vi "NACA_0015_Pressure_with_profile_fixed.vi"(3 "Mode":T5, 5 "Traverse line In":T1 {"Row Duration (mins)" format="%#.1f"; "Row No" min=0; "Trace Gas Concentration (%)" min=0.0 format="%#.2f"; "Emission Rate (l/min)" format="%#.2f"; "Tunnel Speed" format="%#.2f"; "Start X" format="%#.2f"; "Start Y" format="%#.2f"; "Start Z" format="%#.2f"; "End X" format="%#.2f"; "End Y" format="%#.2f"; "End Z" format="%#.2f"; "Averaging time (min)" min=0.0 format="%#.2f"}) -> (0 "Error Message":string, 1 "Status":T4, 2 "Traverse line Out":T1 {"Row Duration (mins)" format="%#.1f"; "Row No" min=0; "Trace Gas Concentration (%)" min=0.0 format="%#.2f"; "Emission Rate (l/min)" format="%#.2f"; "Tunnel Speed" format="%#.2f"; "Start X" format="%#.2f"; "Start Y" format="%#.2f"; "Start Z" format="%#.2f"; "End X" format="%#.2f"; "End Y" format="%#.2f"; "End Z" format="%#.2f"; "Averaging time (min)" min=0.0 format="%#.2f"})   [LabVIEW 2012]
uses:
  Gen Trav/Traverse_cluster.ctl
  Gen Trav/Spacing.ctl
  Controls/Multi_run_mode.ctl
  Controls/User_Specific_mode.ctl
  Gen Trav/Multi_Run_Status.ctl
  Gen Trav/Trav_mode.ctl
  Controls/Setup.ctl
  Controls/Save_Data.ctl
  <vilib>/Analysis/1siggen.llb/Ramp Pattern by Delta.vi
  <vilib>/Analysis/1siggen.llb/Ramp Pattern by Samples.vi
  Globals/Extra_Commands_Global.vi
  Globals/Meas_global.vi
  <vilib>/Analysis/NI_AALBase.lvlib
panel:
  out "Wake Profile":cluster{dbl[], dbl[]}(graph)
  in  "stop":bool
  out "Pressure":cluster{dbl[], dbl[]}(graph)
  out "Measurement No":i32
  # "X           Y            Z"
  # "Start"
  # "End"
  # "X           Y            Z"
  # "Start"
  # "End"
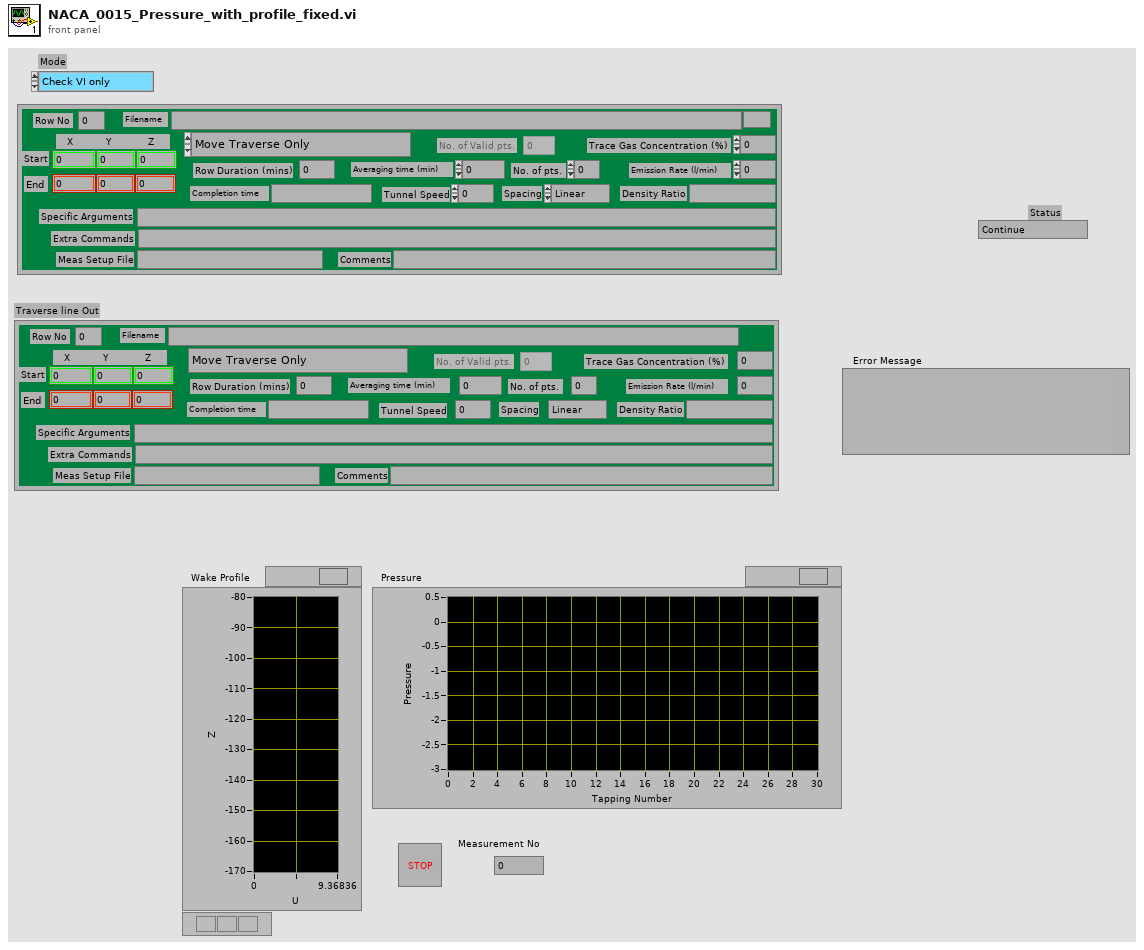
[diagram p1: front panel]
types:
  T1 = typedef "Traverse_cluster.ctl" = cluster{"Start X":dbl, "Start Y":dbl, "Start Z":dbl, "End X":dbl, "End Y":dbl, "End Z":dbl, "No. of pts.":i32, "Spacing":T2, "Filename":path, "Tunnel Speed":dbl, "Averaging time (min)":dbl, "Extra Commands":string, "Specific Arguments":string, "Emission Rate (l/min)":dbl, "Trace Gas Concentration (%)":dbl, "Density Ratio":string, "Comments":string, "Row No":i32, "Row Type Selector":T3, "Completion time":string, "Row Duration (mins)":dbl, "No. of Valid pts.":i32, "Meas Setup File":string}
  T2 = typedef "Spacing.ctl" = enum16{"Linear", "Log", "Gauss", "Specified", "N/A"}
  T3 = typedef "Multi_run_mode.ctl" = enum16{"Move Traverse Only", "Set Tunnel Speed Only", "Set Source Only", "Set Measurement Conditions", "Single Measurement", "Vertical Profile", "Lateral Profile", "Longitudinal Profile", "Explore Volume", "Multi-Axis Profile", "Auto Calibrate", "Meas Fast FID Bkgnd", "Check Beam Power", "Scanning Valve Measurement", "Run VI Named:", "Set ADAM Ch", "Wait (minutes)", "Send Message", "Synchronize With:", "Fall Back to this Row", "Turn Off Row Repeating", "Blank Row", "Traverse 3D Volume"}
  T4 = typedef "Multi_Run_Status.ctl" = enum16{"Continue", "Jump to Next Point", "Jump to Next Row", "Jump To Fall Back", "Terminate Run"}
  T5 = typedef "User_Specific_mode.ctl" = enum16{"Check VI only", "Run VI"}
  T6 = typedef "Trav_mode.ctl" = enum16{"Move traverse", "Read traverse position", "Teach Position"}
  T7 = typedef "Save_Data.ctl" = enum16{"Save No Data", "Save Data"}
  T8 = typedef "Setup.ctl" = enum16{"Run Program", "Show Setup", "Save Current Setup", "Setup Front Panel"}
  T9 = typedef "Status_Cluster.ctl" = cluster{"Status":T4, "Error Type":string, "Error Description":string}
  T10 = typedef "Analysis_info_cluster.ctl" = cluster{"Colour":u32, "Inst type":T11, "Inst name":string, "Symbol":string, "Code name":string, "Extra Info":string, "Inst Array":T12, "Extra Titles":string[], "Extra Values":string[], "U":dbl, "u^2":dbl, "u^3":dbl, "u^4":dbl, "Skew_u":dbl, "Kurt_u":dbl, "Sd Error in Mean":dbl, "% u'/U":dbl, "X":dbl, "Y":dbl, "Z":dbl, "Timescale integral to 25%":dbl, "Sd Error in Variance":dbl, "Calib File":path, "Calib Constants":dbl[], "Output Position":bool, "Full Stats":bool, "Av Sampling Rate":dbl, "Av No of Samples":dbl, "Total Meas Time (s)":dbl, "ADAM Ch Name":string}
  T11 = typedef "Inst_type.ctl" = enum16{"Propeller anemometer", "Raw voltage", "Pressure Transducer", "Pitot-static tube", "Preston tube", "Hot wire", "Cross wire 1", "Cross wire 2", "Generic Linear", "Generic Polynomial", "Generic BackPoly", "Fast FID", "Thermocouple", "Cold wire", "Pulsed Wire", "LDA Vel", "LDA Tran time", "LDA Arr time"}
  T12 = typedef "Instrument_Array.ctl" = enum16{"PWA", "LDA", "Analogue"}
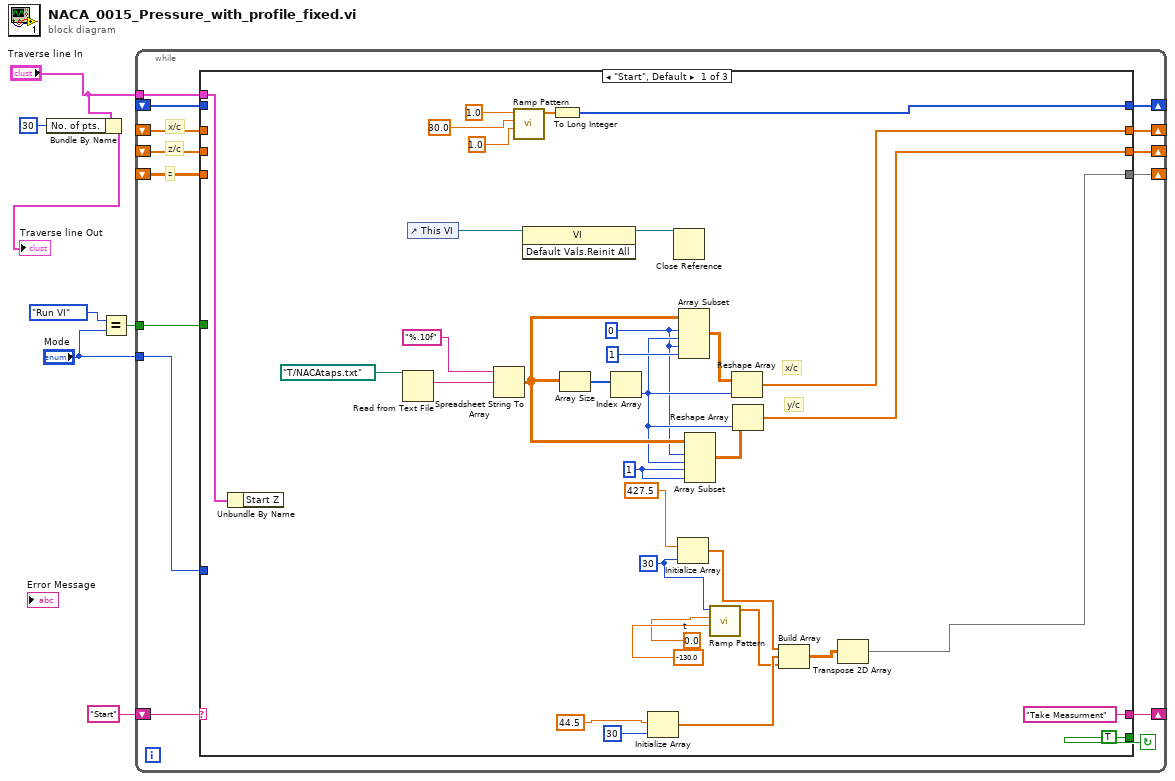
[diagram p0: block diagram]
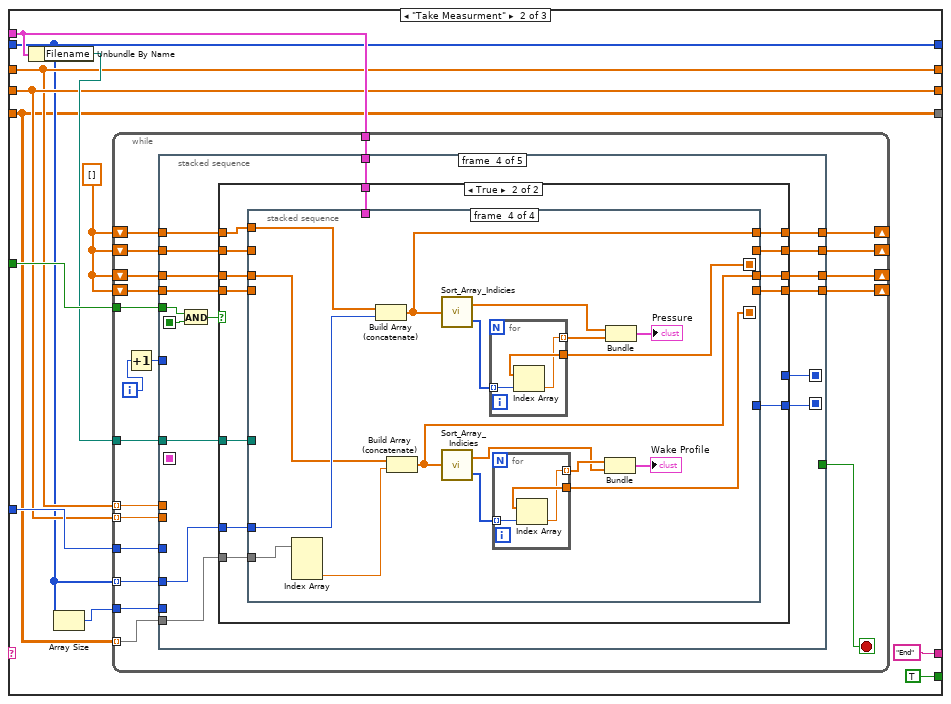
[diagram p2: hidden frame]
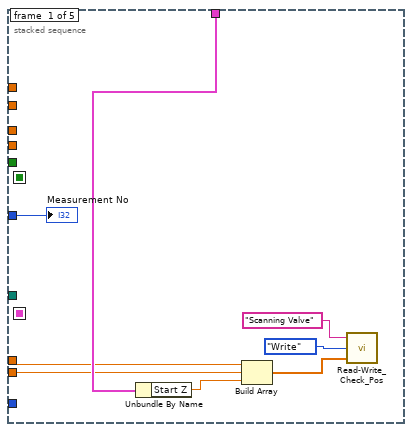
[diagram p3: hidden frame]
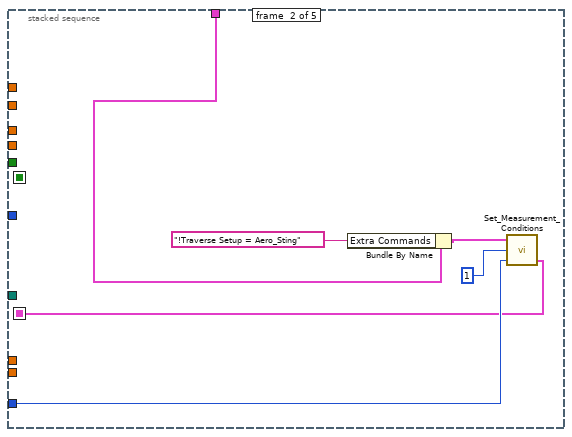
[diagram p4: hidden frame]
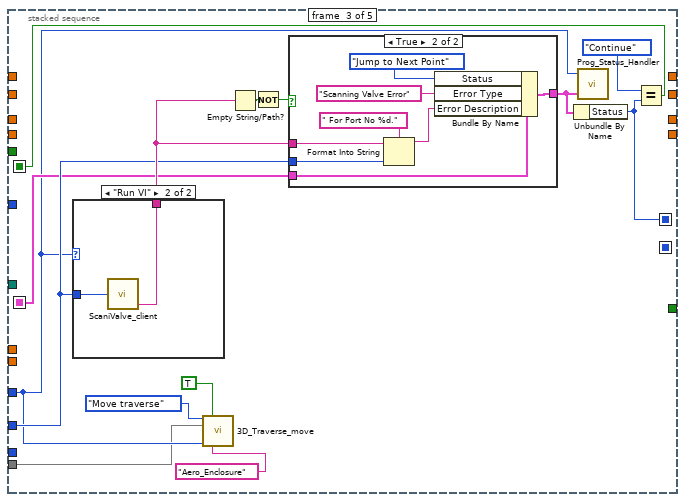
[diagram p5: hidden frame]
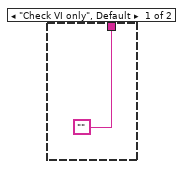
[diagram p6: hidden frame]
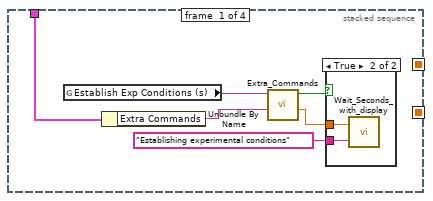
[diagram p9: hidden frame]
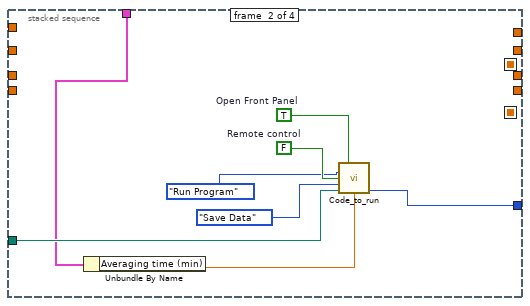
[diagram p11: hidden frame]
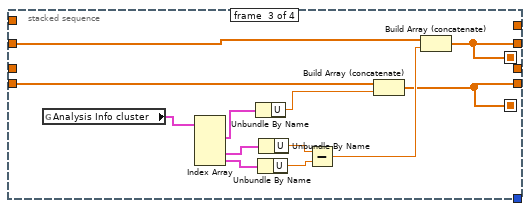
[diagram p12: hidden frame]
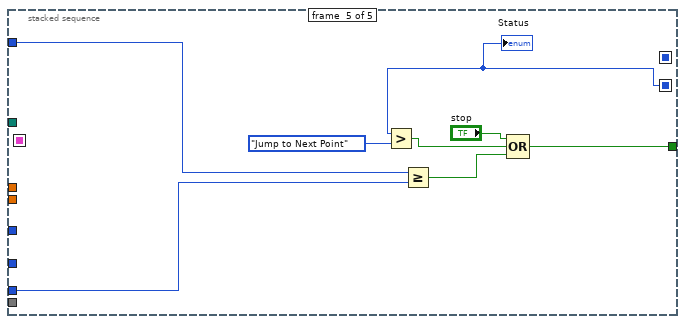
[diagram p13: hidden frame]
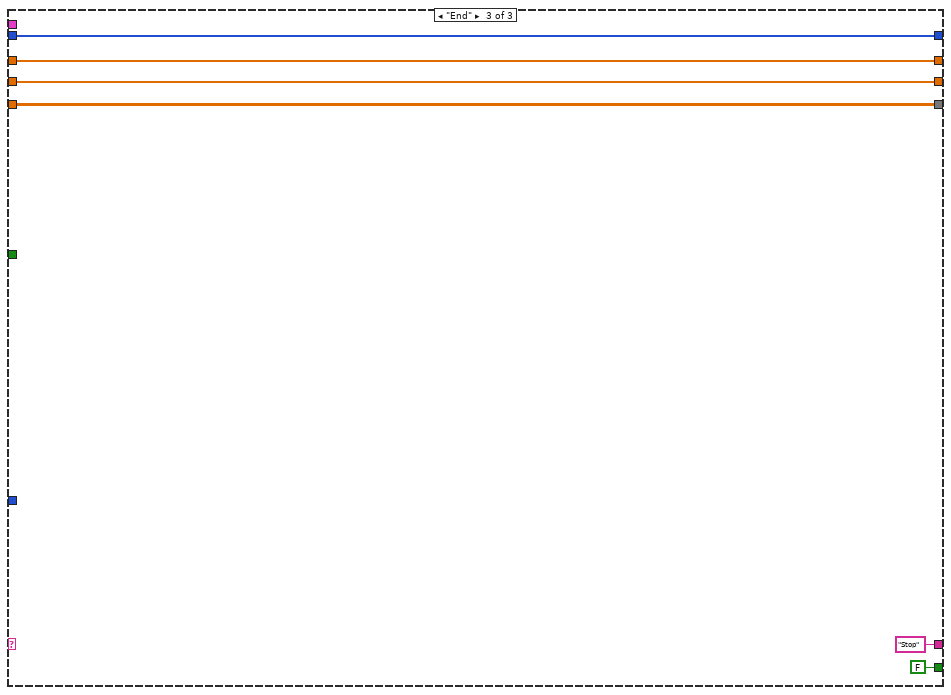
[diagram p14: hidden frame]
diagram:
  n1 = Bundle By Name(cluster="Traverse line In", "No. of pts."=30) -> (→"Traverse line Out":T1)
  n2 = Equal?(x=User_Specific_mode."Run VI" ("Mode"), y="Mode") -> (x = y?=w4:bool)
  n3 = while {
    tunnel: "Traverse line In" -> [w20]
    shift-right: [w19] -> _
    shift-left: "Start" -> [w18]
    tunnel: "Mode" -> [w17]
    tunnel: w4 -> [w16]
    shift-right: [w15] -> _
    shift-left: _ -> [w14]
    shift-right: [w13] -> _
    shift-left: _ -> [w11]
    shift-right: [w12] -> _
    shift-left: _ -> [w10]
    shift-right: [w9] -> _
    shift-left: _ -> [w8]
    stop <- w21 continue-if-true
    # "z"
    # "z/c"
    # "x/c"
    n4 = case shown="\"Start\", Default" w18 {
      tunnel: [TRUE TRUE FALSE] -> w21
      tunnel: w20 -> [w33 w64 _]
      tunnel: ["Take Measurment" "End" "Stop"] -> w19
      tunnel: w17 -> [_ w62 _]
      tunnel: w16 -> [_ w65 _]
      tunnel: [w51 w59 w225] -> w15
      tunnel: w14 -> [_ w59 w225]
      tunnel: [w37 w60 w224] -> w13
      tunnel: [w36 w61 w223] -> w12
      tunnel: w11 -> [_ w60 w224]
      tunnel: w10 -> [_ w61 w223]
      tunnel: [w23 w57 w222] -> w9
      tunnel: w8 -> [_ w57 w222]
      frame "Start", Default {
        w32 = 30 ("samples")
        w22 = 0.0  # t
        w38 = 1 ("index")
        w39 = 0 ("index")
        # "y/c"
        # "x/c"
        n5 = Unbundle By Name(w33) -> ()  [unwired: 1 out]
        n6 = Read from Text File(file (use dialog)=path "T:/NACAtaps.txt") -> (text=w47:string)  [unwired: 3 in, 3 out]
        n7 = control-ref of="This VI"() -> (w35:refnum<vi>)
        n8 = Spreadsheet String To Array(format string="%.10f", spreadsheet string=w47) -> (array=w43:dbl[][])  [unwired: 2 in]
        n9 = call-poly <vilib>:"Ramp Pattern.vi"("start"=1.0, "end"=30.0, "delta"=1.0) -> ("Ramp Pattern"=w55:dbl[])  [unwired: 6 in, 2 out]
        n10 = invoke class="VI" method="Default Vals.Reinit All"(reference=w35) -> (reference out=w34:refnum<vi>)  [unwired: 2 in, 2 out]
        n11 = To Long Integer(number=w55) -> (32bit integer=w51:i32[])
        n12 = Array Size(array=w43) -> (size(s)=w45:i32[])
        n13 = Index Array(array=w45) -> (element=w40:i32)  [unwired: 1 in]
        n14 = Initialize Array(44.5 ("Y"), 30 ("dimension size")) -> (w27:dbl[])
        n15 = Close Reference(reference=w34) -> ()  [unwired: 1 in, 1 out]
        n16 = Initialize Array(427.5 ("X"), w32) -> (w25:dbl[])
        n17 = Array Subset(array=w43, index (row)=w39, length (row)=w40, index (col)=w39, length (col)=1 ("length")) -> (w42:dbl[][])
        n18 = Array Subset(array=w43, index (row)=w39, length (row)=w40, index (col)=w38, length (col)=w38) -> (w41:dbl[][])
        n19 = call-poly <vilib>:"Ramp Pattern.vi"("start"=-130.0, "end"=w22, "samples"=w32) -> ("Ramp Pattern"=w26:dbl[])  [unwired: 7 in, 1 out]
        n20 = Reshape Array(w42, w40) -> (w37:dbl[])
        n21 = Reshape Array(w41, w40) -> (w36:dbl[])
        n22 = Build Array(w25, w27, w26) -> (w24:dbl[][])
        n23 = Transpose 2D Array(2D array=w24) -> (transposed array=w23:dbl[][])
      }
      frame "Take Measurment" {
        w56 = dbl[] []
        n24 = Unbundle By Name(w64) -> ("Filename"=w63:path)
        n25 = Array Size(array=w59) -> (size(s)=w58:i32)
        n26 = while {
          tunnel: w62 -> [w82]
          tunnel: w65 -> [w79]
          tunnel: w63 -> [w87]
          shift-right: [w85] -> _
          shift-left: w56 -> [w86]
          shift-right: [w83] -> _
          shift-left: w56 -> [w84]
          tunnel: w64 -> [w81]
          tunnel: w59 -> [w76] mode=indexing
          tunnel: w60 -> [w75] mode=indexing
          tunnel: w61 -> [w74] mode=indexing
          tunnel: w58 -> [w73]
          tunnel: w57 -> [w72] mode=indexing
          shift-right: [w71] -> _
          shift-left: w56 -> [w70]
          shift-right: [w68] -> _
          shift-left: w56 -> [w69]
          i -> [w78]
          stop <- w80 stop-if-true
          n27 = Increment(x=w78) -> (x+1=w77:i32)
          n28 = stacked-sequence {
            seq-local: [_ _ w110 _ _] -> [_ _ _ w136 _]
            seq-local: [_ _ w109 _ _] -> [_ _ _ w137 _]
            seq-local: [_ _ _ w138 _] -> [_ _ _ _ w215]
            seq-local: [_ w96 _ _ _] -> [_ _ w107 _ _]
            tunnel: w87 -> [_ _ _ w144 _]
            tunnel: w86 -> [_ _ _ w143 _]
            tunnel: [_ _ _ w142 _] -> w85
            tunnel: w84 -> [_ _ _ w141 _]
            tunnel: [_ _ _ w140 _] -> w83
            tunnel: w82 -> [_ w97 w105 _ _]
            tunnel: w81 -> [w94 w98 _ w139 _]
            tunnel: w77 -> [w95 _ _ _ w218]
            tunnel: [_ _ _ _ w216] -> w80
            tunnel: w79 -> [_ _ _ w135 _]
            tunnel: w76 -> [_ _ w108 w133 _]
            tunnel: w75 -> [w93 _ _ _ _]
            tunnel: w74 -> [w92 _ _ _ _]
            tunnel: w73 -> [_ _ _ _ w214]
            tunnel: w72 -> [_ _ w102 w132 _]
            tunnel: [_ _ _ w131 _] -> w71
            tunnel: w70 -> [_ _ _ w130 _]
            tunnel: w69 -> [_ _ _ w129 _]
            tunnel: [_ _ _ w128 _] -> w68
            frame #0 {
              n29 = Unbundle By Name(w94) -> ("Start Z"=w91:dbl)
              n30 = Build Array(w93, w92, w91) -> (w90:dbl[])
              n31 = call "Read-Write_Check_Pos.vi"("Position input"=w90, "Mode"=enum16{"Read", "Write"}."Write", "Traverse Name"="Scanning Valve") -> ()  [unwired: 1 out]
              "Measurement No" <- w95
            }
            frame #1 {
              n32 = Bundle By Name(cluster=w98, "Extra Commands"="!Traverse Setup = Aero_Sting") -> (w101:T1)
              n33 = call "Set_Measurement_Conditions.vi"("Simulate/Run"=w97, "Currently on Point"=1, "Traverse line"=w101) -> ("Status Cluster"=w96:T9)  [unwired: 2 in]
            }
            frame #2 {
              n34 = case shown="\"Run VI\"" w105 {
                tunnel: w108 -> [_ w118]
                tunnel: ["" w117] -> w113
                frame "Check VI only", Default {
                }
                frame "Run VI" {
                  n35 = call "ScaniValve_client.vi"("Port Number"=w118) -> ("Error String"=w117:string)  [unwired: 2 out]
                }
              }
              n36 = call "3D_Traverse_move.vi"("Mode"=Trav_mode."Move traverse", "Route Checking?"=TRUE, "Position"=w102, "Simulate/Run"=w105, "Traverse name"="Aero_Enclosure" ("Traverse Name")) -> ()  [unwired: 8 in, 3 out]
              n37 = Empty String/Path?(string/path=w113) -> (empty?=w115:bool)
              n38 = Not(x=w115) -> (.not. x?=w114:bool)
              n39 = case shown="True" w114 {
                tunnel: w107 -> [w119 w127]
                tunnel: [w119 w124] -> w111
                tunnel: w113 -> [_ w121]
                tunnel: w108 -> [_ w120]
                frame False {
                }
                frame True {
                  n40 = Format Into String(format string=" For Port No %d." ("Format String"), initial string=w121, w120) -> (resulting string=w122:string)  [unwired: 1 in, 1 out]
                  n41 = Bundle By Name(cluster=w127, "Status"=Multi_Run_Status."Jump to Next Point", "Error Type"="Scanning Valve Error" ("t"), "Error Description"=w122) -> (w124:T9)
                }
              }
              n42 = Unbundle By Name(w111) -> ("Status"=w109:T4)
              n43 = call "Prog_Status_Handler.vi"("Status Cluster"=w111, "Simulate/Run"=w105) -> ()  [unwired: 2 out]
              n44 = Equal?(x=Multi_Run_Status."Continue" ("Status"), y=w109) -> (x = y?=w110:bool)
            }
            frame #3 {
              n45 = And(x=w135, y=w136) -> (x .and. y?=w134:bool)
              n46 = case shown="True" w134 {
                tunnel: [w147 w162] -> w138
                tunnel: w144 -> [_ w161]
                tunnel: w143 -> [w149 w160]
                tunnel: [w149 w159] -> w142
                tunnel: w141 -> [w148 w158]
                tunnel: [w148 w157] -> w140
                tunnel: w139 -> [_ w156]
                tunnel: w133 -> [_ w155]
                tunnel: w137 -> [w147 _]
                tunnel: w132 -> [_ w154]
                tunnel: [w145 w153] -> w131
                tunnel: w130 -> [w145 w152]
                tunnel: w129 -> [w146 w151]
                tunnel: [w146 w150] -> w128
                frame False {
                }
                frame True {
                  n47 = stacked-sequence {
                    seq-local: [_ _ w189 _] -> [_ _ _ w202]
                    seq-local: [_ _ w180 _] -> [_ _ _ w197]
                    tunnel: [_ w173 _ _] -> w162
                    tunnel: w161 -> [_ w172 _ _]
                    tunnel: w160 -> [_ _ w190 _]
                    tunnel: [_ _ w189 _] -> w159
                    tunnel: w158 -> [_ _ _ w207]
                    tunnel: [_ _ _ w205] -> w157
                    tunnel: w156 -> [w168 w171 _ _]
                    tunnel: w155 -> [_ _ _ w200]
                    tunnel: w154 -> [_ _ _ w199]
                    tunnel: [_ _ w180 _] -> w153
                    tunnel: w152 -> [_ _ w179 _]
                    tunnel: w151 -> [_ _ _ w192]
                    tunnel: [_ _ _ w191] -> w150
                    frame #0 {
                      n48 = global read "Extra_Commands_Global.vi" "Establish Exp Conditions (s)"() -> (w165:string)
                      n49 = Unbundle By Name(w168) -> ("Extra Commands"=w167:string)
                      n50 = call "Extra_Commands.vi"("String to Search"=w167, "Command"=w165) -> ("Numeric Value"=w166:dbl, "Command Found"=w164:bool)  [unwired: 2 in, 2 out]
                      n51 = case shown="True" w164 {
                        tunnel: w166 -> [_ w170]
                        tunnel: "Establishing experimental conditions" ("Message") -> [_ w169]
                        frame False {
                        }
                        frame True {
                          n52 = call "Wait_Seconds_with_display.vi"("Message"=w169, "Seconds to wait"=w170) -> ()  [unwired: 1 in, 1 out]
                        }
                      }
                    }
                    frame #1 {
                      w176 = TRUE  # Open Front Panel
                      w178 = FALSE  # Remote control
                      n53 = Unbundle By Name(w171) -> ("Averaging time (min)"=w177:dbl)
                      n54 = call "Code_to_run.vi"("Open Front Panel"=w176, "setup"=Setup."Run Program", "Remote control"=w178, "File"=Save_Data."Save Data", "Results Filename"=w172, "Averaging time (min)"=w177) -> ("Status"=w173:T4)  [unwired: 5 in, 4 out]
                    }
                    frame #2 {
                      n55 = global read "Meas_global.vi" "Analysis Info cluster"() -> (w188:T10[])
                      n56 = Index Array(array=w188) -> (element #1=w182:T10, element #3=w183:T10, element #4=w184:T10)  [unwired: 4 in, 1 out]
                      n57 = Unbundle By Name(w182) -> ("U"=w181:dbl)
                      n58 = Unbundle By Name(w184) -> ("U"=w185:dbl)
                      n59 = Unbundle By Name(w183) -> ("U"=w186:dbl)
                      n60 = Subtract(x=w186, y=w185) -> (x-y=w187:dbl)
                      n61 = Build Array (concatenate)(w179, w181) -> (w180:dbl[])
                      n62 = Build Array (concatenate)(w190, w187) -> (w189:dbl[])
                    }
                    frame #3 {
                      n63 = Index Array(array=w199) -> (element #3=w193:dbl)  [unwired: 3 in, 2 out]
                      n64 = Build Array (concatenate)(w207, w200) -> (w205:dbl[])
                      n65 = Build Array (concatenate)(w192, w193) -> (w191:dbl[])
                      n66 = call "Sort_Array_Indicies.vi"("unsorted array"=w205) -> ("sorted array"=w204:dbl[], "Sort Index"=w203:i32[])
                      n67 = call "Sort_Array_Indicies.vi"("unsorted array"=w191) -> ("sorted array"=w194:dbl[], "Sort Index"=w198:i32[])
                      n68 = for {
                        tunnel: w203 -> [w213] mode=indexing
                        tunnel: w202 -> [w212]
                        tunnel: [w211] -> w201 mode=indexing
                        n69 = Index Array(array=w212, index=w213) -> (element=w211:dbl)
                      }
                      n70 = for {
                        tunnel: w198 -> [w210] mode=indexing
                        tunnel: w197 -> [w209]
                        tunnel: [w208] -> w195 mode=indexing
                        n71 = Index Array(array=w209, index=w210) -> (element=w208:dbl)
                      }
                      n72 = Bundle(w195, "sorted array"=w194) -> (→"Wake Profile":cluster{dbl[], "sorted array":dbl[]})  [unwired: 1 out]
                      n73 = Bundle("sorted array"=w204, w201) -> (→"Pressure":cluster{"sorted array":dbl[], dbl[]})  [unwired: 1 out]
                    }
                  }
                }
              }
            }
            frame #4 {
              n74 = Greater?(x=w215, y=Multi_Run_Status."Jump to Next Point" ("Status")) -> (0:w220:bool)
              n75 = Greater Or Equal?(x=w218, y=w214) -> (x >= y?=w219:bool)
              n76 = Compound Arithmetic op=OR("stop", w220, w219) -> (w216:bool)
              "Status" <- w215
            }
          }
        }
      }
      frame "End" {
      }
    }
  }
